vi "PH_PPPA_PowerUnit.PC_StatePSU.vi"(0 "i ref in":refnum<vi>, 3 "State PSU":T1 items=["no info", "off/false/out", "on/true/in", "Failure", "Alarm", "Status 1", "Status 2", "Status 3"], 4 "not linked?":bool, 5 "error in (no error)":errorcluster) -> (14 "i ref out":refnum<vi> caption="VI Refnum", 19 "error out":errorcluster)   [LabVIEW 2014, in "PH_PPPA_PowerUnit.lvlib"]
doc: "This VI writes the PSU Tag Information (Sum Fault and HV on) to own attributes, calculates the state of the device and sets the GUI object."
uses:
  PH_PPPA_PowerUnit.lvlib
  PH_StatusHandler/PH_StatusHandler.Status.ctl
  PH_Common/PH_Common.lvlib
  PH_StatusHandler/PH_StatusHandler.lvlib
  PH_Beckhoff_PP_PU/PH_Beckhoff_PP_PU.lvlib
  PH_PowerUnit_BaseClass/PH_PowerUnit_BaseClass.lvlib
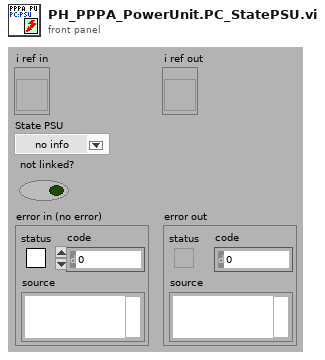
[diagram p1: front panel]
types:
  T1 = typedef "PH_StatusHandler.lvlib/PH_StatusHandler.Status.ctl" = i16
  T2 = typedef "PH_PowerUnit_BaseClass.lvlib/PH_PowerUnit_BaseClass.i attribute.ctl" = cluster{"Constructor finished":bool, "PU":cluster{"In use":bool, "Service ID in use":i32, "GUI Ref":refnum<vi>}, "Enabling":cluster{"State":T3, "GUI Ref":refnum<vi>}, "Timing":cluster{"Last Shot":dbl, "Time between Shots [Sec]":dbl, "Waiting Time over?":bool, "Service ID Waiting Time":i32, "GUI Ref":refnum<vi>, "Instance":cluster{"Status":T1, "linked?":bool, "GUI Ref":refnum<vi>}}, "Sequencer":cluster{"SM State":string, "GUI Ref":refnum<vi>, "linked":bool}, "Subscribed Trendmssgs":cluster{"Tagname":string, "Status":T1, "linked?":bool, "Shot Condition":T1, "GUI Ref":refnum<vi>}[], "PP PU":T4, "Default Voltage (V)":dbl, "GUI Refs":T5, "PSDB data":cluster{"Shot Voltage [V]":dbl, "State TO SM":T6, "Write 2 early":bool}, "State TO SM":T6}
  T3 = typedef "PH_SystemInformation.lvlib/PH_SystemInformationEnabling State.ctl" = i32
  T4 = typedef "PH_PP_Common.lvlib/PH_PP_Common.PUs.ctl" = enum16{"no Info", "PA-19mm-1", "PA-19mm-2", "PA-45mm-PILC", "PA-45mm-MAIN", "MA-PU-1", "MA-PU-2", "MA-PU-3", "MA-PU-4", "MA-PU-5", "MA-PU-6", "MA-FR", "MA-PILC", "PA-45mm-DP"}
  T5 = typedef "PH_PowerUnit_BaseClass.lvlib/PH_PowerUnit_BaseClass.GUI Refs.ctl" = cluster{"Delete Inst":refnum<vi>, "State TO SM":refnum<vi>, "State SM":refnum<vi>, "Fire":refnum<vi>}
  T6 = typedef "PH_PowerUnit_BaseClass.lvlib/PH_PowerUnit_BaseClass.SM States.ctl" = enum16{".", "Stand by", "Switch PU on", "Configure", "Set Default Voltage", "Set STANDBY", "Set READY", "Wait for Shot Cmd", "Open Dump Rods", "Open Ross Relais", "Close Ross Relais", "Switch PSU on", "Switch PSU off", "Charge", "Switch GD Channel on", "Close Dump Rods", "Rods-TO", "RR-TO", "PSU-TO", "Trigger-TO"}
  T7 = typedef "PH_PPPA_PowerUnit.lvlib/PH_PPPA_PowerUnit.i attribute.ctl" = cluster{"GUI Refs":cluster{"Ignitron":refnum<vi>, "Rossrelais":refnum<vi>, "Set Voltage":refnum<vi>, "PSU":refnum<vi>, "EOC":refnum<vi>, "Trigger":refnum<vi>}, "Ignitron":T8, "PSU":T9, "Dump Ross Relais":T10, "Trigger":cluster{"State Device":T1, "linked?":bool}, "Timing Settings":cluster{"Prdc Fast?":bool, "Default Value Periodic Interval":i32, "Mercury on since":dbl, "Warm up Time Mercury [s]":dbl}, "Set Voltage [V]":dbl, "19er Ignitionbox":string}
  T8 = typedef "PH_PP_Common.lvlib/PH_PP_Common.Ignitron Attributes.ctl" = cluster{"State Device":T1, "linked?":bool}
  T9 = typedef "PH_PP_Common.lvlib/PH_PP_Common.PSU Attributes.ctl" = cluster{"lower limit [V]":dbl, "upper limit [V]":dbl, "Voltage set":bool, "State Device":T1, "linked?":bool}
  T10 = typedef "PH_PP_Common.lvlib/PH_PP_Common.Ross Relais Attributes.ctl" = cluster{"State Device":T1, "linked?":bool}
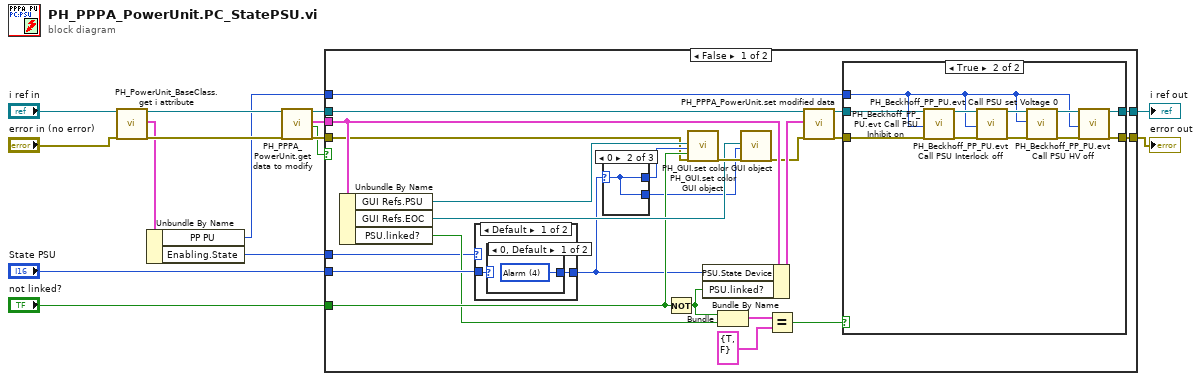
[diagram p0: block diagram]
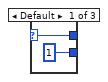
[diagram p2: hidden frame]
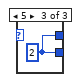
[diagram p3: hidden frame]
diagram:
  n1 = call "PH_PowerUnit_BaseClass.get i attribute.vi"("i ref in"="i ref in", "error in (no error)"="error in (no error)") -> ("i ref out"=w4:refnum<vi>, "i attribute"=w3:T2, "error out"=w6:errorcluster)  [unwired: 15 in]
  n2 = Unbundle By Name(w3) -> ("PP PU"=w1:T4, "Enabling.State"=w2:T3)
  n3 = call "PH_PPPA_PowerUnit.get data to modify.vi"("i ref in"=w4, "error in (no error)"=w6) -> ("i ref out"=w12:refnum<vi>, "i attribute"=w10:T7, "timed out"=w9:bool, "error out"=w11:errorcluster)  [unwired: 14 in]
  n4 = case shown="False" w9 {
    tunnel: w12 -> [w18 w63]
    tunnel: [w21 w63] -> w14
    tunnel: w11 -> [w19 w62]
    tunnel: [w20 w62] -> w15
    tunnel: w10 -> [w37 _]
    tunnel: "State PSU" -> [w36 _]
    tunnel: "not linked?" -> [w30 _]
    tunnel: w2 -> [w17 _]
    tunnel: w1 -> [w16 _]
    frame False {
      n5 = Unbundle By Name(w37) -> ("GUI Refs.PSU"=w32:refnum<vi>, "GUI Refs.EOC"=w31:refnum<vi>, "PSU.linked?"=w29:bool)
      n6 = case shown="Default" w17 {
        tunnel: w36 -> [w58 w61]
        tunnel: [w57 w61] -> w25
        frame Default {
          n7 = case shown="0, Default" w58 {
            selector: w58 -> [_ w60]
            tunnel: [w59 w60] -> w57
            frame 0, Default {
              w59 = T1 4 items=["no info", "off/false/out", "on/true/in", "Failure", "Alarm", "Status 1", "Status 2", "Status 3"] ("PSU.State Device")
            }
            frame 1 {
            }
          }
        }
        frame 1 {
        }
      }
      n8 = case shown="0" w25 {
        selector: w25 -> [w41 w42 _]
        tunnel: [w41 w42 w43] -> w24
        tunnel: [1 ("State") w42 w43] -> w23
        frame Default {
        }
        frame 0 {
        }
        frame 5 {
          w43 = 2 ("State")
        }
      }
      n9 = Not(x=w30) -> (.not. x?=w22:bool)
      n10 = call "PH_GUI.set color GUI object.vi"("GUI object Ref"=w32, "State"=w24, "Blinking? (false)"=w30, "error in (no error)"=w19) -> ("error out"=w38:errorcluster)  [unwired: 15 in]
      n11 = Bundle By Name(cluster=w37, "PSU.State Device"=w25, "PSU.linked?"=w22) -> (w39:T7)
      n12 = Bundle(w22, "linked?"=w29) -> (w28:cluster{bool, "linked?":bool})  [unwired: 1 in]
      n13 = call "PH_GUI.set color GUI object.vi"("GUI object Ref"=w31, "State"=w23, "error in (no error)"=w38) -> ("error out"=w33:errorcluster)  [unwired: 16 in]
      n14 = Equal?(x=w28, y=cluster{"not linked?":bool, "linked?":bool} {"not linked?"=TRUE, "linked?"=FALSE}) -> (x = y?=w26:bool)
      n15 = call "PH_PPPA_PowerUnit.set modified data.vi"("i ref in"=w18, "i attribute"=w39, "error in (no error)"=w33) -> ("i ref out"=w35:refnum<vi>, "error out"=w34:errorcluster)  [unwired: 15 in]
      n16 = case shown="True" w26 {
        tunnel: [w44 w56] -> w20
        tunnel: [w45 w55] -> w21
        tunnel: w35 -> [w45 w46]
        tunnel: w34 -> [w44 w47]
        tunnel: w16 -> [_ w48]
        frame False {
        }
        frame True {
          n17 = call "PH_Beckhoff_PP_PU.evt Call PSU Inhibit on.vi"("i ref in"=w46, "PU"=w48, "error in"=w47) -> ("i ref out"=w52:refnum<vi>, "error out"=w51:errorcluster)  [unwired: 15 in]
          n18 = call "PH_Beckhoff_PP_PU.evt Call PSU Interlock off.vi"("i ref in"=w52, "PU"=w48, "error in"=w51) -> ("i ref out"=w54:refnum<vi>, "error out"=w53:errorcluster)  [unwired: 15 in]
          n19 = call "PH_Beckhoff_PP_PU.evt Call PSU set Voltage 0.vi"("i ref in"=w54, "PU"=w48, "error in"=w53) -> ("i ref out"=w50:refnum<vi>, "error out"=w49:errorcluster)  [unwired: 15 in]
          n20 = call "PH_Beckhoff_PP_PU.evt Call PSU HV off.vi"("i ref in"=w50, "PU"=w48, "error in"=w49) -> ("i ref out"=w55:refnum<vi>, "error out"=w56:errorcluster)  [unwired: 15 in]
        }
      }
    }
    frame True {
    }
  }
  "error out" <- w15
  "i ref out" <- w14
